vi "To String.vi"(11 "JSON Null in":refnum<class "JSON Null.lvclass">) -> (2 "String":string)   [LabVIEW 2017, in "LVJSON.lvlib" / "JSON Null.lvclass"]
uses:
  JSON Null.lvclass
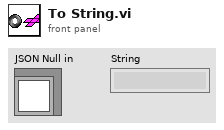
[diagram p1: front panel]
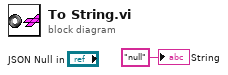
[diagram p0: block diagram]
diagram:
  "String" <- "null" ("String")
